vi "Create Path (string).vi"(5 "URI-Component.Path":refnum<class "URI-Component.Path.lvclass">, 8 "error in (no error)":errorcluster, 10 "base-path":string, 11 "Path":string) -> (0 "error out":errorcluster, 1 "Valid":bool, 2 "Path type":T1=enum."path-abempty", 3 "URI-Component.Path":refnum<class "URI-Component.Path.lvclass">)   [LabVIEW 2013, in "openURI.lvlib" / "URI-Component.Path.lvclass"]
uses:
  URI-Component.Path.lvclass
  path type -- enum.ctl
  URI-Component.Path.lvclass/URI-Component.Path.ctl
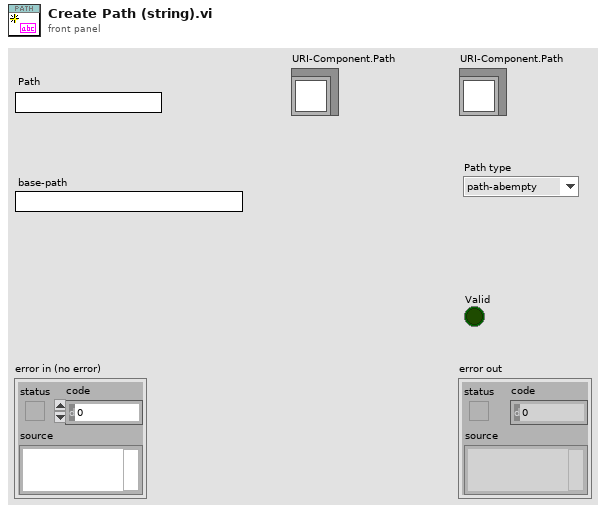
[diagram p1: front panel]
types:
  T1 = typedef "openURI.lvlib/URI-Component.Path.lvclass/path type -- enum.ctl" = enum16{"invalid", "path-abempty", "path-absolute", "path-noscheme", "path-rootless", "path-empty"}
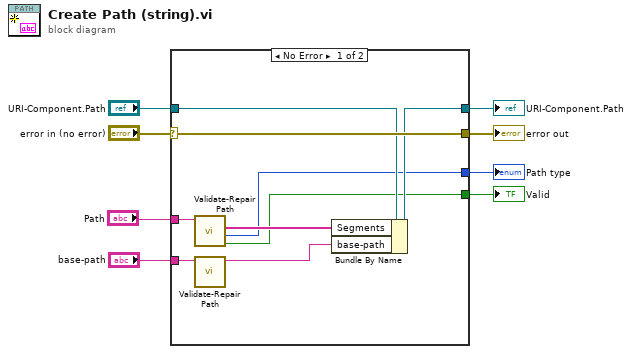
[diagram p0: block diagram]
diagram:
  n1 = case shown="No Error" "error in (no error)" {
    selector: "error in (no error)" -> [w17 w19]
    tunnel: [w17 w19] -> w7
    tunnel: [w15 w18] -> w5
    tunnel: "URI-Component.Path" -> [w16 w18]
    tunnel: "Path" -> [w12 _]
    tunnel: [w10 _] -> w3
    tunnel: [w9 _] -> w2
    tunnel: "base-path" -> [w14 _]
    frame No Error {
      n2 = call "Validate-Repair Path.vi"("path in"=w12) -> ("Valid"=w9:bool, "Path type"=w10:T1, "Segments"=w11:string[])  [unwired: 7 in, 1 out]
      n3 = call "Validate-Repair Path.vi"("path in"=w14) -> ("path out"=w13:string)  [unwired: 7 in, 3 out]
      n4 = Bundle By Name(cluster=w16, "Segments"=w11, "base-path"=w13) -> (w15:refnum<class "URI-Component.Path.lvclass">)
    }
    frame Error {
    }
  }
  "error out" <- w7
  "URI-Component.Path" <- w5
  "Valid" <- w2
  "Path type" <- w3
